vi "Get Property.vi"(10 "Ctl Ref":refnum<vi>, 11 "ValueUIP In":refnum<class "ValueUIP.lvclass">) -> (0 "Error Out":errorcluster, 3 "ValueUIP Out":refnum<class "ValueUIP.lvclass">)   [LabVIEW 2015, in "ValueUIP.lvclass"]
doc: "Overwrite this abstract method to implement child behavior for getting the property from the VI Server Control and into the UIP private data."
uses:
  ValueUIP.lvclass
  ValueUIP.lvclass/ValueUIP.ctl
  <vilib>/Utility/Data Type/NI_Data Type.lvlib
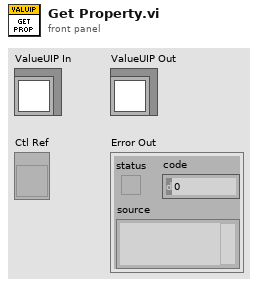
[diagram p1: front panel]
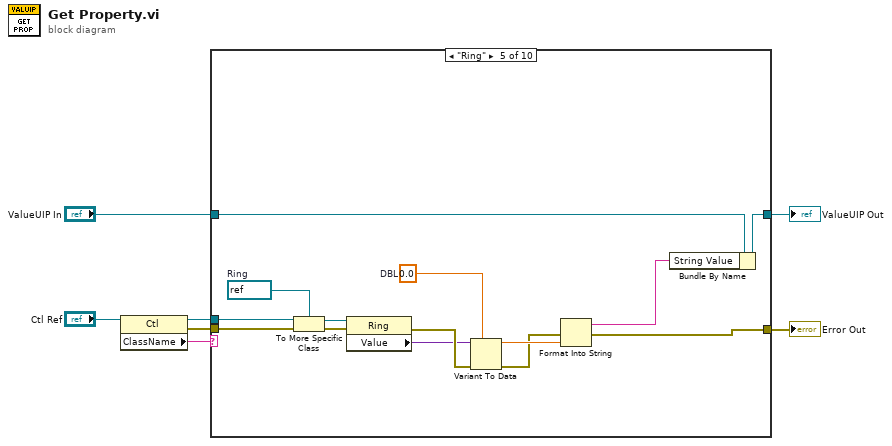
[diagram p0: block diagram]
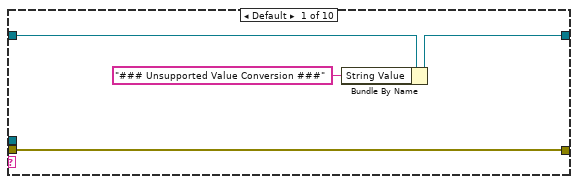
[diagram p2: hidden frame]
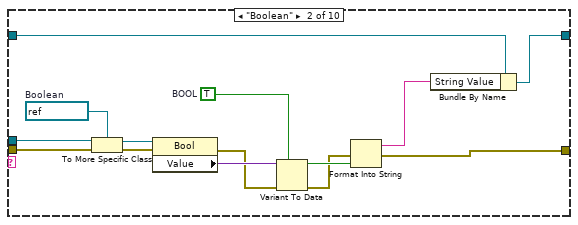
[diagram p3: hidden frame]
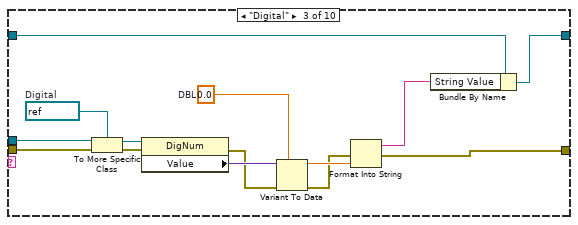
[diagram p4: hidden frame]
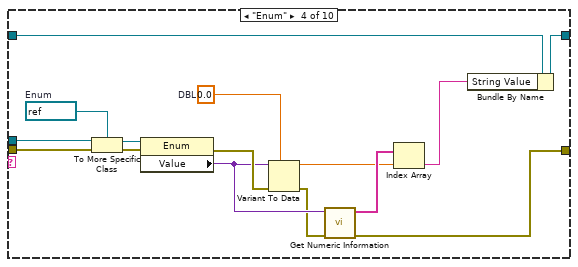
[diagram p5: hidden frame]
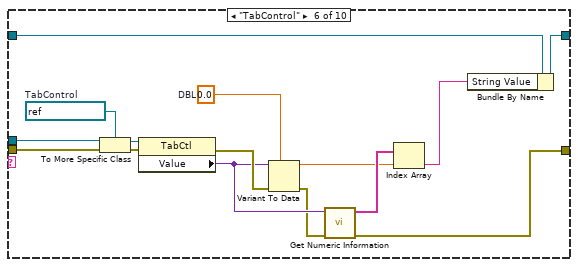
[diagram p6: hidden frame]
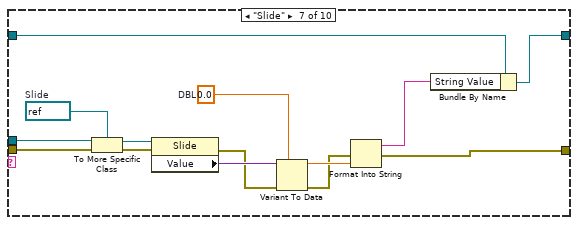
[diagram p7: hidden frame]
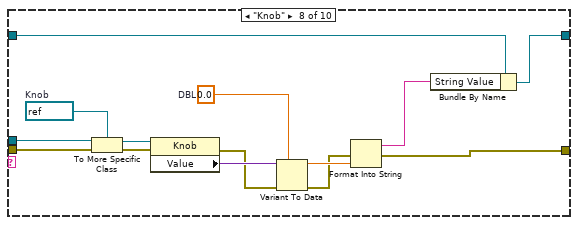
[diagram p8: hidden frame]
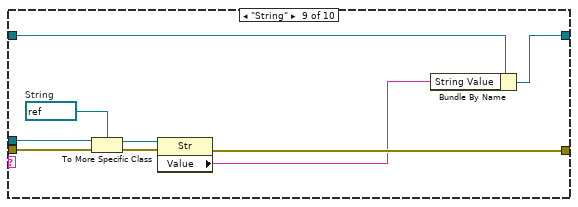
[diagram p9: hidden frame]
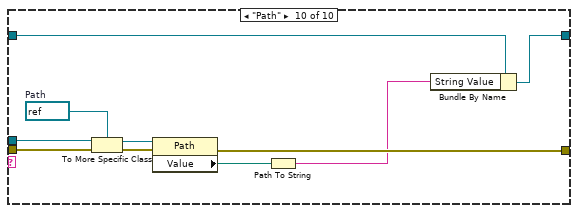
[diagram p10: hidden frame]
diagram:
  n1 = property class="Ctl"(reference="Ctl Ref") -> (reference out=w6:refnum<vi>, error out=w5:errorcluster, "ClassName"=w7:string)  [unwired: 1 in]
  n2 = case shown="\"Ring\"" w7 {
    tunnel: w6 -> [_ w25 w39 w54 w68 w83 w97 w111 w120 w130]
    tunnel: w5 -> [w11 w24 w38 w53 w67 w82 w96 w110 w119 w129]
    tunnel: "ValueUIP In" -> [w10 w15 w29 w47 w61 w76 w87 w101 w115 w125]
    tunnel: [w9 w14 w28 w46 w60 w75 w86 w100 w114 w124] -> w3
    tunnel: [w11 w12 w26 w40 w56 w69 w84 w98 w113 w123] -> w2
    frame Default {
      n3 = Bundle By Name(cluster=w10, "String Value"="### Unsupported Value Conversion ###") -> (w9:refnum<class "ValueUIP.lvclass">)
    }
    frame "Boolean" {
      w18 = TRUE  # BOOL
      w23 = refnum<vi> refnum  # Boolean
      n4 = To More Specific Class(target class=w23, reference=w25, error in=w24) -> (specific class reference=w22:refnum<vi>, error out=w21:errorcluster)
      n5 = property class="Bool"(reference=w22, error in=w21) -> (error out=w19:errorcluster, "Value"=w20:variant)  [unwired: 1 out]
      n6 = Variant To Data(error in=w19, type=w18, Variant=w20) -> (data=w17:bool, error out=w16:errorcluster)
      n7 = Format Into String(error in=w16, w17) -> (resulting string=w13:string, error out=w12:errorcluster)  [unwired: 2 in]
      n8 = Bundle By Name(cluster=w15, "String Value"=w13) -> (w14:refnum<class "ValueUIP.lvclass">)
    }
    frame "Digital" {
      w32 = 0.0  # DBL
      w37 = refnum<vi> refnum  # Digital
      n9 = To More Specific Class(target class=w37, reference=w39, error in=w38) -> (specific class reference=w36:refnum<vi>, error out=w35:errorcluster)
      n10 = property class="DigNum"(reference=w36, error in=w35) -> (error out=w33:errorcluster, "Value"=w34:variant)  [unwired: 1 out]
      n11 = Variant To Data(error in=w33, type=w32, Variant=w34) -> (data=w31:dbl, error out=w30:errorcluster)
      n12 = Format Into String(error in=w30, w31) -> (resulting string=w27:string, error out=w26:errorcluster)  [unwired: 2 in]
      n13 = Bundle By Name(cluster=w29, "String Value"=w27) -> (w28:refnum<class "ValueUIP.lvclass">)
    }
    frame "Enum" {
      w48 = 0.0  # DBL
      w52 = refnum<vi> refnum  # Enum
      n14 = To More Specific Class(target class=w52, reference=w54, error in=w53) -> (specific class reference=w51:refnum<vi>, error out=w50:errorcluster)
      n15 = property class="Enum"(reference=w51, error in=w50) -> (error out=w49:errorcluster, "Value"=w45:variant)  [unwired: 1 out]
      n16 = Variant To Data(error in=w49, type=w48, Variant=w45) -> (data=w43:dbl, error out=w41:errorcluster)
      n17 = call <vilib>:"Get Numeric Information.vi"("error in (no error)"=w41, "Variant"=w45) -> ("error out"=w40:errorcluster, "Enum Names"=w44:string[])  [unwired: 6 in, 2 out]
      n18 = Index Array(array=w44, index=w43) -> (element=w42:string)
      n19 = Bundle By Name(cluster=w47, "String Value"=w42) -> (w46:refnum<class "ValueUIP.lvclass">)
    }
    frame "Ring" {
      w62 = 0.0  # DBL
      w66 = refnum<vi> refnum  # Ring
      n20 = To More Specific Class(target class=w66, reference=w68, error in=w67) -> (specific class reference=w65:refnum<vi>, error out=w64:errorcluster)
      n21 = property class="Ring"(reference=w65, error in=w64) -> (error out=w63:errorcluster, "Value"=w59:variant)  [unwired: 1 out]
      n22 = Variant To Data(error in=w63, type=w62, Variant=w59) -> (data=w58:dbl, error out=w57:errorcluster)
      n23 = Format Into String(error in=w57, w58) -> (resulting string=w55:string, error out=w56:errorcluster)  [unwired: 2 in]
      n24 = Bundle By Name(cluster=w61, "String Value"=w55) -> (w60:refnum<class "ValueUIP.lvclass">)
    }
    frame "TabControl" {
      w77 = 0.0  # DBL
      w81 = refnum<vi> refnum  # TabControl
      n25 = To More Specific Class(target class=w81, reference=w83, error in=w82) -> (specific class reference=w80:refnum<vi>, error out=w79:errorcluster)
      n26 = property class="TabCtl"(reference=w80, error in=w79) -> (error out=w78:errorcluster, "Value"=w74:variant)  [unwired: 1 out]
      n27 = Variant To Data(error in=w78, type=w77, Variant=w74) -> (data=w72:dbl, error out=w70:errorcluster)
      n28 = call <vilib>:"Get Numeric Information.vi"("error in (no error)"=w70, "Variant"=w74) -> ("error out"=w69:errorcluster, "Enum Names"=w73:string[])  [unwired: 6 in, 2 out]
      n29 = Index Array(array=w73, index=w72) -> (element=w71:string)
      n30 = Bundle By Name(cluster=w76, "String Value"=w71) -> (w75:refnum<class "ValueUIP.lvclass">)
    }
    frame "Slide" {
      w90 = 0.0  # DBL
      w95 = refnum<vi> refnum  # Slide
      n31 = To More Specific Class(target class=w95, reference=w97, error in=w96) -> (specific class reference=w94:refnum<vi>, error out=w93:errorcluster)
      n32 = property class="Slide"(reference=w94, error in=w93) -> (error out=w91:errorcluster, "Value"=w92:variant)  [unwired: 1 out]
      n33 = Variant To Data(error in=w91, type=w90, Variant=w92) -> (data=w89:dbl, error out=w88:errorcluster)
      n34 = Format Into String(error in=w88, w89) -> (resulting string=w85:string, error out=w84:errorcluster)  [unwired: 2 in]
      n35 = Bundle By Name(cluster=w87, "String Value"=w85) -> (w86:refnum<class "ValueUIP.lvclass">)
    }
    frame "Knob" {
      w104 = 0.0  # DBL
      w109 = refnum<vi> refnum  # Knob
      n36 = To More Specific Class(target class=w109, reference=w111, error in=w110) -> (specific class reference=w108:refnum<vi>, error out=w107:errorcluster)
      n37 = property class="Knob"(reference=w108, error in=w107) -> (error out=w105:errorcluster, "Value"=w106:variant)  [unwired: 1 out]
      n38 = Variant To Data(error in=w105, type=w104, Variant=w106) -> (data=w103:dbl, error out=w102:errorcluster)
      n39 = Format Into String(error in=w102, w103) -> (resulting string=w99:string, error out=w98:errorcluster)  [unwired: 2 in]
      n40 = Bundle By Name(cluster=w101, "String Value"=w99) -> (w100:refnum<class "ValueUIP.lvclass">)
    }
    frame "String" {
      w118 = refnum<vi> refnum  # String
      n41 = To More Specific Class(target class=w118, reference=w120, error in=w119) -> (specific class reference=w117:refnum<vi>, error out=w116:errorcluster)
      n42 = property class="Str"(reference=w117, error in=w116) -> (error out=w113:errorcluster, "Value"=w112:string)  [unwired: 1 out]
      n43 = Bundle By Name(cluster=w115, "String Value"=w112) -> (w114:refnum<class "ValueUIP.lvclass">)
    }
    frame "Path" {
      w128 = refnum<vi> refnum  # Path
      n44 = To More Specific Class(target class=w128, reference=w130, error in=w129) -> (specific class reference=w127:refnum<vi>, error out=w126:errorcluster)
      n45 = property class="Path"(reference=w127, error in=w126) -> (error out=w123:errorcluster, "Value"=w122:path)  [unwired: 1 out]
      n46 = Path To String(path=w122) -> (string=w121:string)
      n47 = Bundle By Name(cluster=w125, "String Value"=w121) -> (w124:refnum<class "ValueUIP.lvclass">)
    }
  }
  "Error Out" <- w2
  "ValueUIP Out" <- w3
